vi "sub_TabloBoya_Flicker.vi"(2 "Table in":refnum<vi>, 3 "Tablo Degerleri":dbl[][](array[numeric])) -> (0 "Test Result":bool, 1 "RESULTS":string[](array[string]))   [LabVIEW 2014]
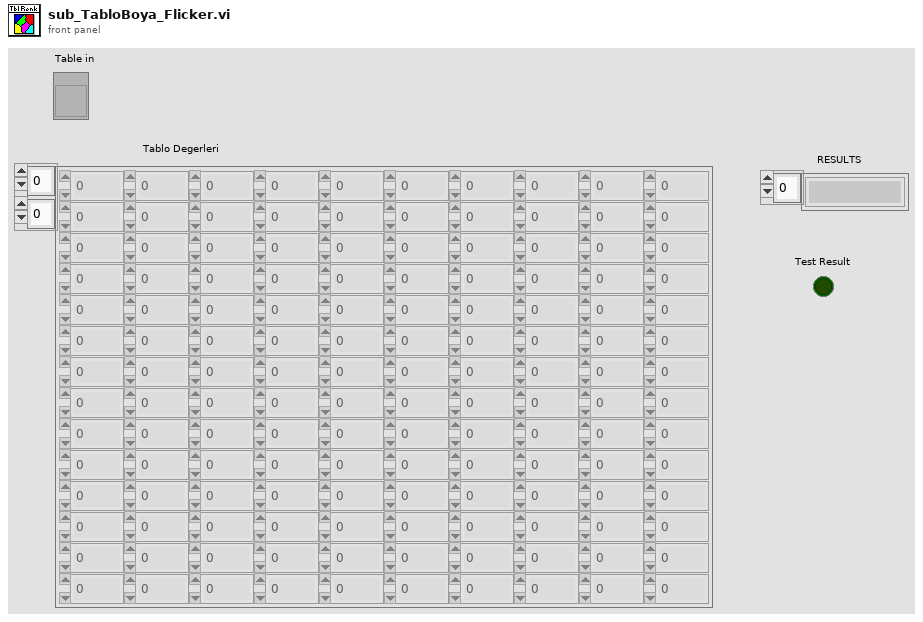
[diagram p1: front panel]
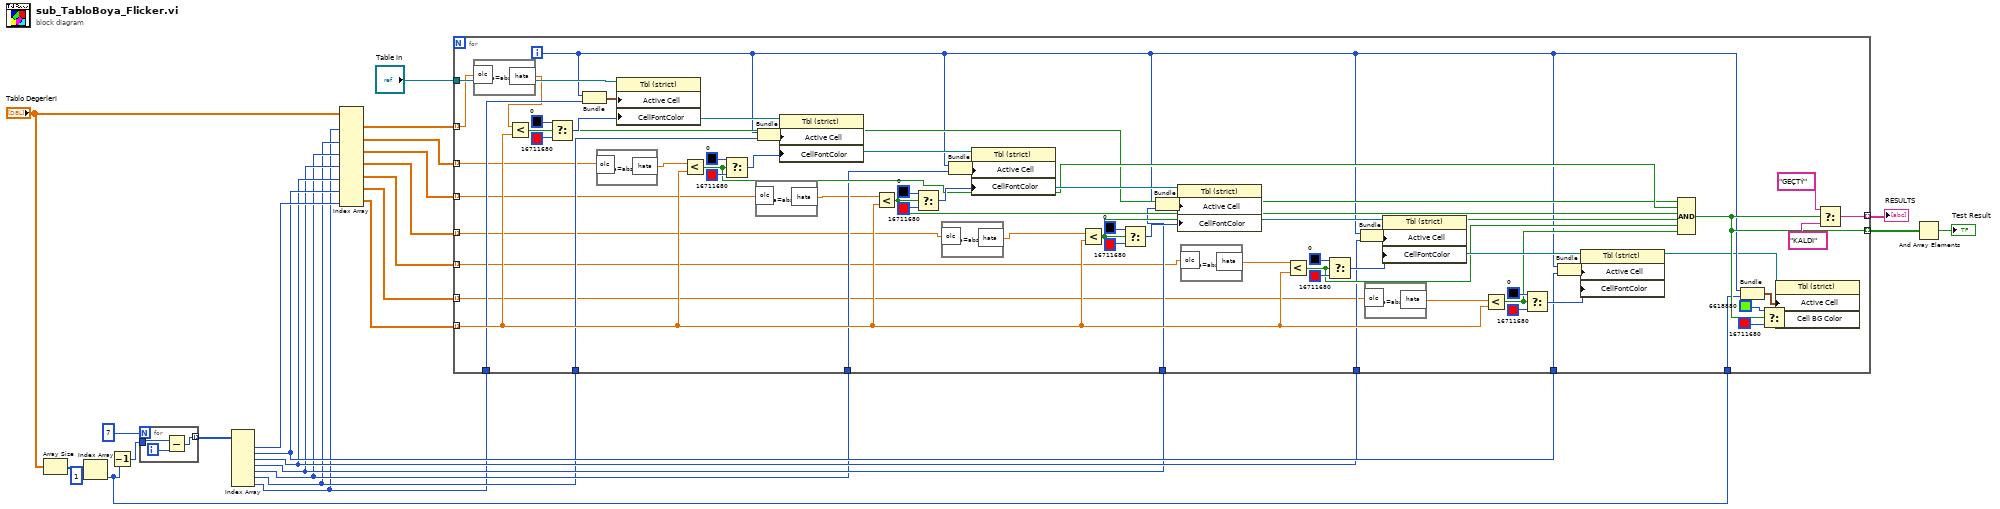
[diagram p0: block diagram]
diagram:
  n1 = Array Size(array="Tablo Degerleri") -> (size(s)=w13:i32[])
  n2 = Index Array(array=w13, index=1) -> (element=w7:i32)
  n3 = Decrement(x=w7) -> (x-1=w8:i32)
  n4 = for {
    N: 7 -> [_]
    tunnel: [w26] -> w11 mode=indexing
    tunnel: w8 -> [w27]
    i -> [w28]
    n5 = Subtract(x=w27, y=w28) -> (x-y=w26:i32)
  }
  n6 = Index Array(array=w11) -> (element #1=w9:i32, element #2=w6:i32, element #3=w5:i32, element #4=w4:i32, element #5=w3:i32, element #6=w2:i32, element #7=w1:i32)  [unwired: 7 in]
  n7 = Index Array(array="Tablo Degerleri", index (col) #1=w1, index (col) #2=w2, index (col) #3=w3, index (col) #4=w4, index (col) #5=w5, index (col) #6=w6, index (col) #7=w9) -> (element #1=w23:dbl[], element #2=w22:dbl[], element #3=w24:dbl[], element #4=w21:dbl[], element #5=w20:dbl[], element #6=w19:dbl[], element #7=w18:dbl[])  [unwired: 7 in]
  n8 = for {
    tunnel: "Table in" -> [w91]
    tunnel: w24 -> [w36] mode=indexing
    tunnel: w23 -> [w38] mode=indexing
    tunnel: w22 -> [w40] mode=indexing
    tunnel: w21 -> [w33] mode=indexing
    tunnel: w20 -> [w31] mode=indexing
    tunnel: w19 -> [w29] mode=indexing
    tunnel: w18 -> [w64] mode=indexing
    tunnel: [w55] -> w17 mode=indexing
    tunnel: [w54] -> w16 mode=indexing
    tunnel: w7 -> [w47]
    tunnel: w6 -> [w46]
    tunnel: w5 -> [w45]
    tunnel: w4 -> [w44]
    tunnel: w3 -> [w43]
    tunnel: w2 -> [w41]
    tunnel: w1 -> [w42]
    i -> [w50]
    n9 = formula code="hata=abs(olc-1);"("olc"=w38) -> ("hata"=w37:dbl)
    n10 = Less?(x=w37, y=w64) -> (x < y?=w58:bool)
    n11 = Select(t=u32 0, s=w58, f=u32 16711680) -> (s? t:f=w92:u32)
    n12 = Bundle(w50, w42) -> (w90:cluster{i32, i32})  [unwired: 1 in]
    n13 = formula code="hata=abs(olc-1);"("olc"=w40) -> ("hata"=w39:dbl)
    n14 = property on="Property Node" class="Tbl (strict)"(reference=w91, "Active Cell"=w90, "CellFontColor"=w92) -> (reference out=w85:refnum<vi>)  [unwired: 1 in, 1 out]
    n15 = Less?(x=w39, y=w64) -> (x < y?=w59:bool)
    n16 = Select(t=u32 0, s=w59, f=u32 16711680) -> (s? t:f=w88:u32)
    n17 = formula code="hata=abs(olc-1);"("olc"=w36) -> ("hata"=w35:dbl)
    n18 = Bundle(w50, w41) -> (w89:cluster{i32, i32})  [unwired: 1 in]
    n19 = property on="Property Node" class="Tbl (strict)"(reference=w85, "Active Cell"=w89, "CellFontColor"=w88) -> (reference out=w80:refnum<vi>)  [unwired: 1 in, 1 out]
    n20 = Less?(x=w35, y=w64) -> (x < y?=w60:bool)
    n21 = Select(t=u32 0, s=w60, f=u32 16711680) -> (s? t:f=w82:u32)
    n22 = formula code="hata=abs(olc-1);"("olc"=w33) -> ("hata"=w34:dbl)
    n23 = Bundle(w50, w43) -> (w81:cluster{i32, i32})  [unwired: 1 in]
    n24 = property on="Property Node" class="Tbl (strict)"(reference=w80, "Active Cell"=w81, "CellFontColor"=w82) -> (reference out=w75:refnum<vi>)  [unwired: 1 in, 1 out]
    n25 = Less?(x=w34, y=w64) -> (x < y?=w61:bool)
    n26 = Select(t=u32 0, s=w61, f=u32 16711680) -> (s? t:f=w77:u32)
    n27 = Bundle(w50, w44) -> (w76:cluster{i32, i32})  [unwired: 1 in]
    n28 = property on="Property Node" class="Tbl (strict)"(reference=w75, "Active Cell"=w76, "CellFontColor"=w77) -> (reference out=w70:refnum<vi>)  [unwired: 1 in, 1 out]
    n29 = formula code="hata=abs(olc-1);"("olc"=w31) -> ("hata"=w32:dbl)
    n30 = Less?(x=w32, y=w64) -> (x < y?=w62:bool)
    n31 = Select(t=u32 0, s=w62, f=u32 16711680) -> (s? t:f=w72:u32)
    n32 = Bundle(w50, w45) -> (w71:cluster{i32, i32})  [unwired: 1 in]
    n33 = formula code="hata=abs(olc-1);"("olc"=w29) -> ("hata"=w30:dbl)
    n34 = property on="Property Node" class="Tbl (strict)"(reference=w70, "Active Cell"=w71, "CellFontColor"=w72) -> (reference out=w65:refnum<vi>)  [unwired: 1 in, 1 out]
    n35 = Less?(x=w30, y=w64) -> (x < y?=w63:bool)
    n36 = Select(t=u32 0, s=w63, f=u32 16711680) -> (s? t:f=w67:u32)
    n37 = Bundle(w50, w46) -> (w66:cluster{i32, i32})  [unwired: 1 in]
    n38 = property on="Property Node" class="Tbl (strict)"(reference=w65, "Active Cell"=w66, "CellFontColor"=w67) -> (reference out=w48:refnum<vi>)  [unwired: 1 in, 1 out]
    n39 = Compound Arithmetic op=AND(w58, w59, w60, w61, w62, w63) -> (w54:bool)
    n40 = Bundle(w50, w47) -> (w49:cluster{i32, i32})  [unwired: 1 in]
    n41 = Select(t=u32 6618880, s=w54, f=u32 16711680) -> (s? t:f=w51:u32)
    n42 = property on="Property Node" class="Tbl (strict)"(reference=w48, "Active Cell"=w49, "Cell BG Color"=w51) -> ()  [unwired: 1 in, 2 out]
    n43 = Select(t="GEÇTÝ", s=w54, f="KALDI") -> (s? t:f=w55:string)
  }
  "RESULTS" <- w17
  n44 = And Array Elements(Boolean array=w16) -> (logical AND=→"Test Result":bool)
